vi "Power Supply.vi"(8 "error in (no error)":errorcluster, 11 "Power Supply in":refnum<class "Power Supply.lvclass">) -> (0 "error out":errorcluster, 3 "Power Supply out":refnum<class "Power Supply.lvclass">)   [LabVIEW 2009, in "Power Supply.lvclass"]
uses:
  Power Supply.lvclass
  Global/GPIB Numbers.vi
  Power Supply.lvclass/Power Supply.ctl
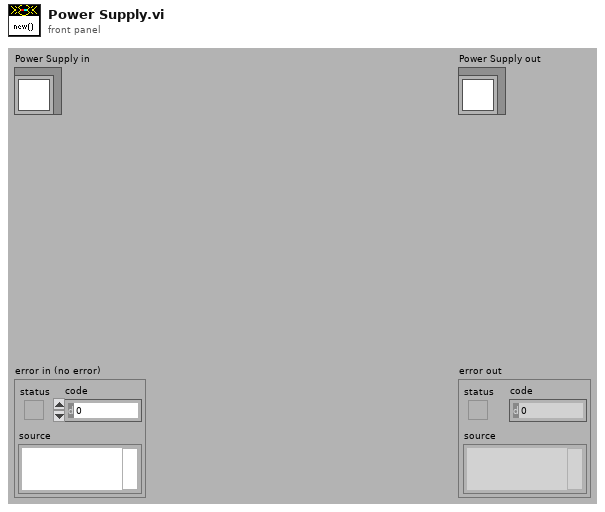
[diagram p1: front panel]
types:
  T1 = typedef "PSIO.ctl" = cluster{"Address":T2, "Version":enum16{"PS", "IPS"}}
  T2 = typedef "OxfordAddress.ctl" = cluster{"Com Port":i32, "ISOBUS Address":i32, "GPIB Address":i16, "Communication":enum16{"RS232", "ISOBUS", "GPIB", "Gateway"}}
  T3 = cluster{"Address":T2, "ILM Name":string, "Display Channel":i32[]}
  T4 = typedef "GPIB Type Def.ctl" = cluster{"Name":string, "bus":dbl, "GPIB":dbl, "GPIB as string":string, "byte":i32, "VISA Resource Name":refnum<visa-resource-name>}
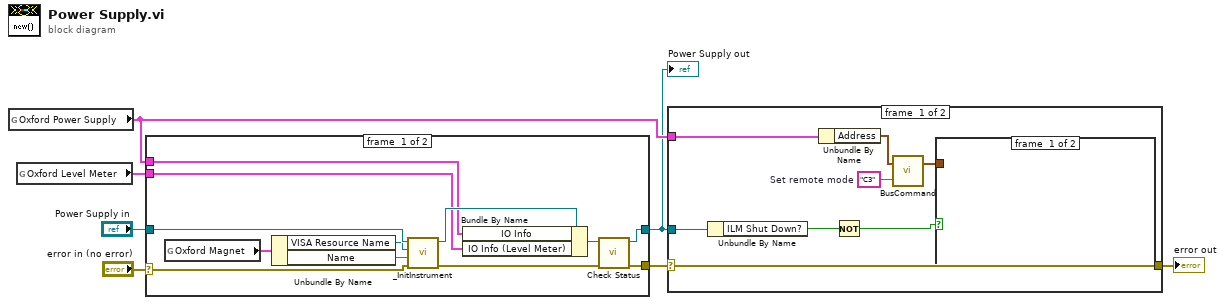
[diagram p0: block diagram]
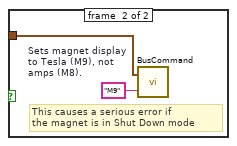
[diagram p2: hidden frame]
diagram:
  n1 = global read "GPIB Numbers.vi" "Oxford Power Supply"() -> (w5:T1)
  n2 = global read "GPIB Numbers.vi" "Oxford Level Meter"() -> (w2:T3)
  n3 = case shown="No Error" "error in (no error)" {
    selector: "error in (no error)" -> [w13 w21]
    tunnel: [w10 w21] -> w4
    tunnel: [w12 w20] -> w1
    tunnel: "Power Supply in" -> [w19 w20]
    tunnel: w5 -> [w9 _]
    tunnel: w2 -> [w8 _]
    frame #0 {
      n4 = global read "GPIB Numbers.vi" "Oxford Magnet"() -> (w16:T4)
      n5 = Unbundle By Name(w16) -> ("VISA Resource Name"=w15:refnum<visa-resource-name>, "Name"=w14:string)
      n6 = call-dynamic "_InitInstrument.vi"("error in (no error)"=w13, "Name"=w14, "VISA Resource Name"=w15, "Instrument in"=w19) -> ("error out"=w11:errorcluster, "Instrument out"=w17:refnum<class "Power Supply.lvclass">)  [unwired: 6 in]
      n7 = Bundle By Name(cluster=w17, "IO Info"=w9, "IO Info (Level Meter)"=w8) -> (w18:refnum<class "Power Supply.lvclass">)
      n8 = call-dynamic "Check Status.vi"("error in (no error)"=w11, "Power Supply in"=w18) -> ("error out"=w10:errorcluster, "Power Supply out"=w12:refnum<class "Power Supply.lvclass">)  [unwired: 6 in, 2 out]
    }
    frame #1 {
    }
  }
  "Power Supply out" <- w1
  n9 = case shown="No Error" w4 {
    selector: w4 -> [w25 w32]
    tunnel: w5 -> [w26 _]
    tunnel: [w25 w32] -> w3
    tunnel: w1 -> [w24 _]
    frame #0 {
      w28 = "C3"  # Set remote mode
      n10 = Unbundle By Name(w24) -> ("ILM Shut Down?"=w23:bool)
      n11 = Unbundle By Name(w26) -> ("Address"=w27:T2)
      n12 = Not(x=w23) -> (.not. x?=w22:bool)
      n13 = call "BusCommand.vi"("Command"=w28, "Instrument address (in)"=w27) -> ("Instrument address (out)"=w29:T2)  [unwired: 1 out]
      n14 = case shown="True" w22 {
        tunnel: w29 -> [_ w31]
        frame #0 {
        }
        frame #1 {
          w30 = "M9"  # Sets magnet display to Tesla (M9), not  amps (M8).
          # "This causes a serious error if \nthe magnet is in Shut Down mode"
          n15 = call "BusCommand.vi"("Command"=w30, "Instrument address (in)"=w31) -> ()  [unwired: 2 out]
        }
      }
    }
    frame #1 {
    }
  }
  "error out" <- w3
